vi "Elapsed Time.vi"(10 "reset timer":bool) -> (0 "elapsed time (s)":dbl, 1 "start time":timestamp, 2 "current time":timestamp)   [LabVIEW 2021, in "Interval Timer.lvlib"]
uses:
  Interval Timer.lvlib
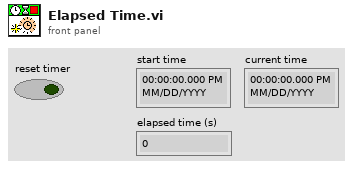
[diagram p1: front panel]
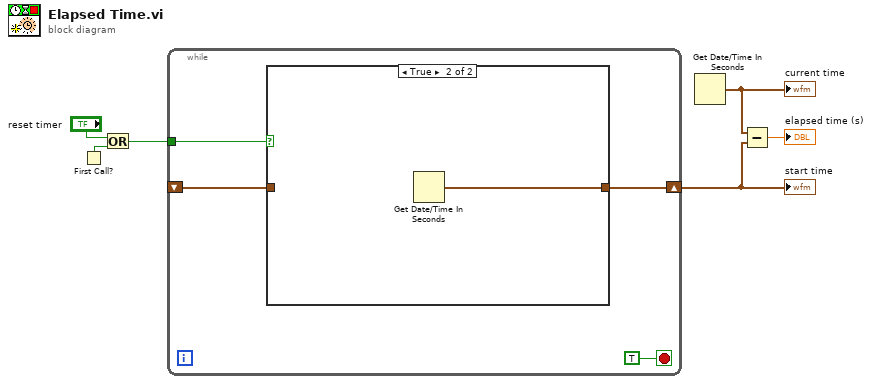
[diagram p0: block diagram]
diagram:
  n1 = First Call?() -> (First Call?: T/F=w5:bool)
  n2 = Or(x="reset timer", y=w5) -> (x .or. y?=w4:bool)
  n3 = while {
    tunnel: w4 -> [w9]
    shift-right: [w8] -> w3
    shift-left: _ -> [w7]
    stop <- TRUE stop-if-true
    n4 = case shown="True" w9 {
      tunnel: [w11 w12] -> w8
      tunnel: w7 -> [w11 _]
      frame False {
      }
      frame True {
        n5 = Get Date/Time In Seconds() -> (seconds since 1Jan1904=w12:timestamp)
      }
    }
  }
  "start time" <- w3
  n6 = Get Date/Time In Seconds() -> (seconds since 1Jan1904=w2:timestamp)
  "current time" <- w2
  n7 = Subtract(x=w2, y=w3) -> (x-y=→"elapsed time (s)":dbl)
